vi "Remote Island.vi"(8 "error in":errorcluster, 11 "Master Controller in":refnum<class "EMS User Interface.lvclass">) -> (0 "error out":errorcluster, 3 "Master Controller out":refnum<class "EMS User Interface.lvclass">)   [LabVIEW 2018, in "EMS User Interface Actor.lvlib" / "EMS User Interface.lvclass"]
uses:
  EMS User Interface.lvclass
  EMS User Interface.lvclass/EMS User Interface.ctl
  <vilib>/ActorFramework/Message Enqueuer/Message Enqueuer.lvclass/Message Enqueuer.ctl
  <vilib>/ActorFramework/Message Enqueuer/Enqueue.vi
  EMS Core/EMS Messages/Island Init Msg/Island Init Msg.lvclass
  C:/Program Files (x86)/National Instruments/LabVIEW 2018/vi.lib/ActorFramework/Message/Message.lvclass
  <vilib>/ActorFramework/Message Priority Queue/Priority Enqueue.vi
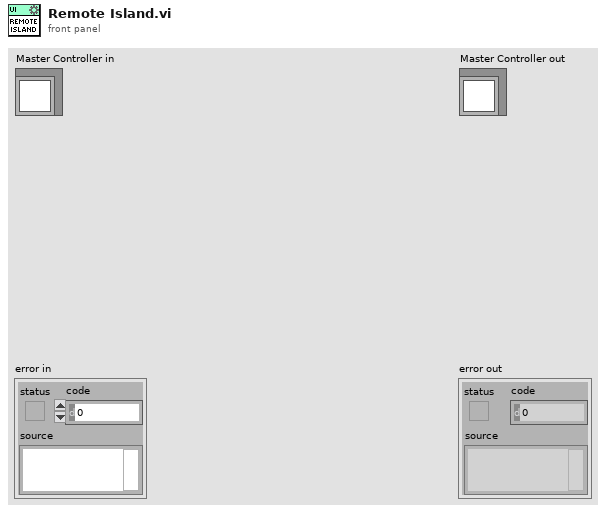
[diagram p1: front panel]
types:
  T1 = typedef "EMS Core.lvlib/EMS.lvclass/Microgrid State.ctl" = enum16{"Discovery", "Commissioning", "Activation", "Blackstart", "OnGrid", "OffGrid", "Island", "Resynchronization", "Manual", "Shutdown", "Stop"}
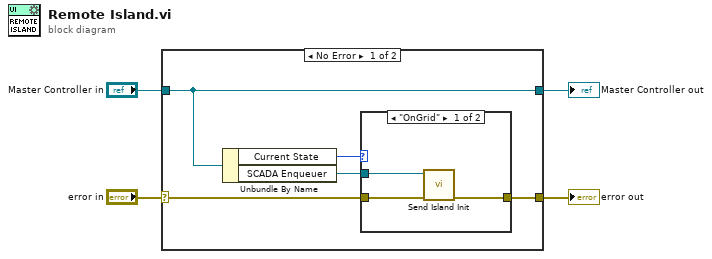
[diagram p0: block diagram]
diagram:
  n1 = case shown="No Error" "error in" {
    selector: "error in" -> [w6 w15]
    tunnel: [w5 w15] -> w2
    tunnel: [w9 w14] -> w1
    tunnel: "Master Controller in" -> [w9 w14]
    frame No Error {
      n2 = Unbundle By Name(w9) -> ("Current State"=w8:T1, "SCADA Enqueuer"=w7:refnum<class "Message Enqueuer.lvclass">)
      n3 = case shown="\"OnGrid\"" w8 {
        tunnel: w7 -> [w12 _]
        tunnel: w6 -> [w11 w13]
        tunnel: [w10 w13] -> w5
        frame "OnGrid" {
          n4 = call "Send Island Init.vi"("error in (no error)"=w11, "Message Enqueuer"=w12) -> ("error out"=w10:errorcluster)  [unwired: 8 in, 1 out]
        }
        frame "Commissioning", Default {
        }
      }
    }
    frame Error {
    }
  }
  "error out" <- w2
  "Master Controller out" <- w1
